vi "Set Visibility.vi"(8 "error in (no error)":errorcluster, 10 "Visible":bool, 11 "GUI Helper in":refnum<class "MessageQ.lvclass">) -> (0 "error out":errorcluster, 3 "GUI Helper out":refnum<class "MessageQ.lvclass">)   [LabVIEW 2020, in "VolatusGUI.lvlib" / "GUI Helper.lvclass"]
uses:
  GUI Helper.lvclass
  Volatus/MessageQ/MessageQ.lvclass
  Visibility Message.ctl
  Volatus/MessageQ/MessageQ.lvclass/MessageQ.ctl
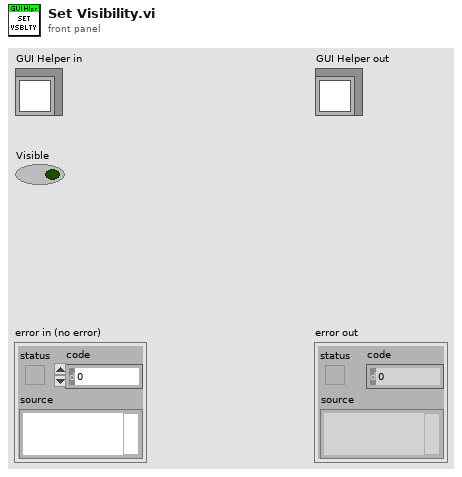
[diagram p1: front panel]
types:
  T1 = typedef "VolatusGUI.lvlib/GUI Helper.lvclass/Visibility Message.ctl" = cluster{"Visible":bool}
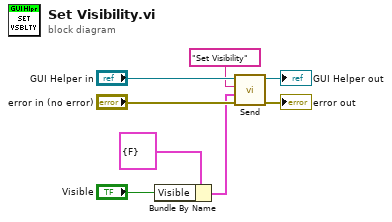
[diagram p0: block diagram]
diagram:
  n1 = Bundle By Name(cluster=T1 {"Visible"=FALSE} ("Visibility Message"), "Visible"="Visible") -> (w2:T1)
  n2 = call "Send.vi"("error in (no error)"="error in (no error)", "Data"=w2, "ID"="Set Visibility", "MessageQ in"="GUI Helper in") -> ("error out"=→"error out":errorcluster, "MessageQ out"=→"GUI Helper out":refnum<class "MessageQ.lvclass">)  [unwired: 6 in]
